vi "parseTemperature.vi"(8 "error in (no error)":errorcluster, 10 "response":string, 11 "XMLResponseParser In":refnum<class "XMLResponseParser.lvclass">) -> (0 "error out":errorcluster, 2 "temperature":i32, 3 "XMLResponseParser Out":refnum<class "XMLResponseParser.lvclass">)   [LabVIEW 2023, in "AbstractFactory.lvlib" / "XMLResponseParser.lvclass"]
uses:
  XMLResponseParser.lvclass
  <vilib>/xml/Close Reference(Node).vi
  XMLResponseParser.lvclass/XMLResponseParser.ctl
  <vilib>/xml/NI_XML.lvlib
  <resource>/objmgr/DOMUserDefRef.rc
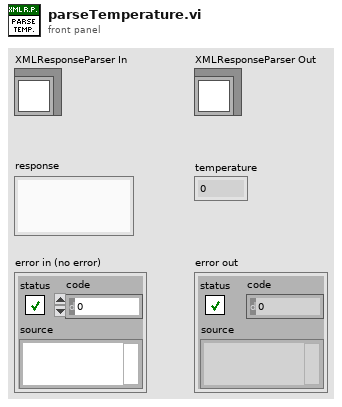
[diagram p1: front panel]
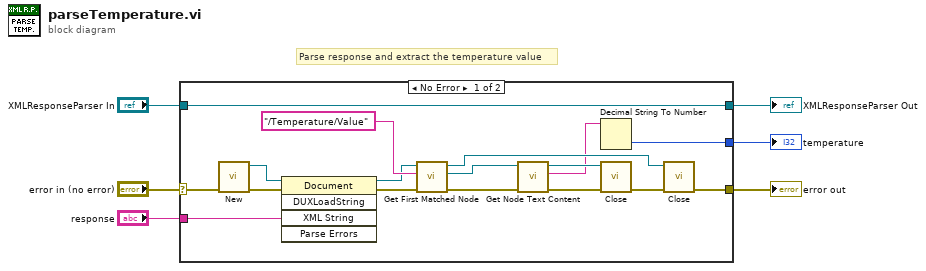
[diagram p0: block diagram]
diagram:
  # "Parse response and extract the temperature value"
  n1 = case shown="No Error" "error in (no error)" {
    selector: "error in (no error)" -> [w19 w25]
    tunnel: [w13 w25] -> w5
    tunnel: [w7 _] -> w4
    tunnel: [w23 w24] -> w2
    tunnel: "XMLResponseParser In" -> [w23 w24]
    tunnel: "response" -> [w21 _]
    frame No Error {
      n2 = call <vilib>:"New.vi"("error in (no error)"=w19) -> ("error out"=w20:errorcluster, "DOM document out"=w22:refnum<k20>)  [unwired: 7 in]
      n3 = invoke class="Document" method="DUXLoadString"(reference=w22, error in=w20, "XML String"=w21) -> (reference out=w16:refnum<k20>, error out=w18:errorcluster)  [unwired: 2 in, 3 out]
      n4 = call <vilib>:"Get First Matched Node.vi"("error in (no error)"=w18, "XPath expression"="/Temperature/Value", "node in"=w16) -> ("error out"=w12:errorcluster, "node result"=w10:refnum<k20>, "node out"=w14:refnum<k20>)  [unwired: 6 in]
      n5 = call <vilib>:"Get Node Text Content.vi"("error in (no error)"=w12, "node in"=w10) -> ("error out"=w11:errorcluster, "node text"=w8:string, "node out"=w9:refnum<k20>)  [unwired: 7 in]
      n6 = Decimal String To Number(string=w8) -> (number=w7:i32)  [unwired: 2 in, 1 out]
      n7 = call-poly <vilib>:"Close.vi"("error in (no error)"=w11, "node"=w9) -> ("error out"=w15:errorcluster)  [unwired: 7 in]
      n8 = call-poly <vilib>:"Close.vi"("error in (no error)"=w15, "node"=w14) -> ("error out"=w13:errorcluster)  [unwired: 7 in]
    }
    frame Error {
    }
  }
  "error out" <- w5
  "XMLResponseParser Out" <- w2
  "temperature" <- w4
